vi "ShooterVI.vi"(0 "Shooter Motor 1":T5={"DeviceStatus"={"status"=FALSE, "code"=0, "source"=""}, "Type"=enum."PWM", "PWM"={"PWM Channel"=enum."PWM 1", "DeadBand"={"Name"="", "maxPositivePwm"=0, "minPositivePwm"=0, "centerPwm"=0, "maxNegativePwm"=0, "minNegativePwm"=0, "angularRange"=0}}, "CAN"={"Device Number"=0, "Control Mode"=enum."Percent VBus", "Semaphore"=refnum, "Max Vout"=12.0, "TalonSRX Control Mode"=enum."Percent VBus"}, "Invert"=FALSE}, 2 "ShooterSolenoid":T3={"DevStatus"={"status"=FALSE, "code"=0, "source"=""}, "Pneumatics Control Module"=0, "Forward Solenoid Channel"=enum."Invalid", "Reverse Solenoid Channel"=enum."Invalid"}, 3 "Roller Angle Motor":T5={"DeviceStatus"={"status"=FALSE, "code"=0, "source"=""}, "Type"=enum."PWM", "PWM"={"PWM Channel"=enum."PWM 1", "DeadBand"={"Name"="", "maxPositivePwm"=0, "minPositivePwm"=0, "centerPwm"=0, "maxNegativePwm"=0, "minNegativePwm"=0, "angularRange"=0}}, "CAN"={"Device Number"=0, "Control Mode"=enum."Percent VBus", "Semaphore"=refnum, "Max Vout"=12.0, "TalonSRX Control Mode"=enum."Percent VBus"}, "Invert"=FALSE}, 5 "Shooter Motor 2":T5={"DeviceStatus"={"status"=FALSE, "code"=0, "source"=""}, "Type"=enum."PWM", "PWM"={"PWM Channel"=enum."PWM 1", "DeadBand"={"Name"="", "maxPositivePwm"=0, "minPositivePwm"=0, "centerPwm"=0, "maxNegativePwm"=0, "minNegativePwm"=0, "angularRange"=0}}, "CAN"={"Device Number"=0, "Control Mode"=enum."Percent VBus", "Semaphore"=refnum, "Max Vout"=12.0, "TalonSRX Control Mode"=enum."Percent VBus"}, "Invert"=FALSE}, 7 "Roller Intake Motor":T5={"DeviceStatus"={"status"=FALSE, "code"=0, "source"=""}, "Type"=enum."PWM", "PWM"={"PWM Channel"=enum."Invalid", "DeadBand"={"Name"="", "maxPositivePwm"=0, "minPositivePwm"=0, "centerPwm"=0, "maxNegativePwm"=0, "minNegativePwm"=0, "angularRange"=0}}, "CAN"={"Device Number"=0, "Control Mode"=enum."Percent VBus", "Semaphore"=refnum, "Max Vout"=12.0, "TalonSRX Control Mode"=enum."Percent VBus"}, "Invert"=FALSE}, 9 "Ball Detector Photoeye":T1, 11 "ShooterAngleMotor":T5={"DeviceStatus"={"status"=FALSE, "code"=0, "source"=""}, "Type"=enum."PWM", "PWM"={"PWM Channel"=enum."PWM 1", "DeadBand"={"Name"="", "maxPositivePwm"=0, "minPositivePwm"=0, "centerPwm"=0, "maxNegativePwm"=0, "minNegativePwm"=0, "angularRange"=0}}, "CAN"={"Device Number"=0, "Control Mode"=enum."Percent VBus", "Semaphore"=refnum, "Max Vout"=12.0, "TalonSRX Control Mode"=enum."Percent VBus"}, "Invert"=FALSE}, 12 "Halo Photoeye":T1, 13 "BallHolderSolenoid":T3={"DevStatus"={"status"=FALSE, "code"=0, "source"=""}, "Pneumatics Control Module"=0, "Forward Solenoid Channel"=enum."Invalid", "Reverse Solenoid Channel"=enum."Invalid"}) -> ()   [LabVIEW 2015]
doc: "This VI controls the shooter, roller intake arm, and shooter angle. It recieves motor references as inputs and runs code in single 100 milisecond metronome loop. Sets PID gains for four PID control loops (two shooter motors, roller intake height, and shooter angle). Runs four state machines, controling the shooter wheels as well as shooter plunger and ball position maintance circle, roller intake position, roller intake PID gains, and shooter angle position."
uses:
  <vilib>/Rock Robotics/WPI/MotorControl/WPI_MotorControlDeviceRef.ctl
  <vilib>/Rock Robotics/WPI/MotorControl/WPI_MotorControlType.ctl
  <vilib>/Rock Robotics/SystemInterfaces/DIO/FPGA_DIOPWMChannel.ctl
  <vilib>/Rock Robotics/WPI/PWM/WPI_PWMDeadband.ctl
  <vilib>/Rock Robotics/WPI/CAN/Jaguar/SubVIs/WPI_CANJaguar_ControlMode.ctl
  <vilib>/Rock Robotics/WPI/CAN/TalonSRX/WPI_CANTalonSRX_APIControlMode.ctl
  <vilib>/Rock Robotics/WPI/DigitalInput/WPI_DigitalInputDevRef.ctl
  <vilib>/Rock Robotics/SystemInterfaces/DIO/FPGA_DIOChannel.ctl
  <vilib>/Rock Robotics/WPI/Solenoid/WPI_SolenoidDevRef.ctl
  <vilib>/Rock Robotics/WPI/Solenoid/WPI_SolenoidChannel.ctl
  <vilib>/Rock Robotics/WPI/DriverStation/WPI_DriverStationRobotMode2.ctl
  <vilib>/Rock Robotics/WPI/Solenoid/WPI_SolenoidValue.ctl
  Team Code/Robot Global Data.vi
  <vilib>/Rock Robotics/Network Tables/NT Write Boolean.vi
  <vilib>/Rock Robotics/WPI/Solenoid/WPI_SolenoidSetEnum.vi
panel:
  in  "Wonder Arm I-Zone 2":dbl=20000.0
  in  "Wonder Arm I 2":dbl=0.0001
  in  "Wonder Arm F 2":dbl
  in  "Wonder Arm D 2":dbl
  in  "Wonder Arm P 2":dbl=0.05
  in  "Wonder Arm Vision Position":dbl=50.0
  in  "Shooter Wheel Gear Ratio":dbl=1.375
  in  "Low Goal Wheel Speed":dbl=-3000.0
  in  "Suck Wheel Speed":dbl=2500.0
  in  "Bumper Shot Wheel Speed":dbl=-3250.0
  in  "High Goal Wheel Speed":dbl=-4500.0
  out "Wonder Arm Angle Throttle":dbl
  in  "Pickup Ball Shooter Angle\n(Competition Bot)":dbl=37.0
  in  "Bumper Shot Shooter Angle\n(Competition Bot)":dbl=8.0
  in  "Low Goal Shooter Angle\n(Competition Bot)":dbl=30.0
  in  "High Goal Shooter Angle\n(Competition Bot)":dbl=17.0
  in  "Shooter Angle Offset":dbl
  in  "Bumper Shot Shooter Angle\n(Practice Bot)":dbl=8.0
  in  "Pickup Ball Shooter Angle\n(Practice Bot)":dbl=37.0
  in  "Low Goal Shooter Angle\n(Practice Bot)":dbl=30.0
  in  "High Goal Shooter Angle\n(Practice Bot)":dbl=17.0
  in  "Wonder Arm Low Bar Position":dbl=60.0
  in  "Wonder Arm Down Position":dbl=58.0
  in  "Wonder Arm Pickup Ball Position":dbl=45.0
  in  "Wonder Arm Up Position":dbl
  out "Shooter Angle Throttle":dbl
  in  "Wonder Arm I-Zone":dbl
  in  "Wonder Arm I":dbl
  in  "Wonder Arm F":dbl
  in  "Wonder Arm D":dbl
  in  "Wonder Arm P":dbl=0.01
  out "Shooter Angle Encoder Value":dbl
  out "Shooter Angle Sensor Position":dbl
  in  "Shooter Angle I-Zone":dbl=4000.0
  in  "Shooter Angle I":dbl=1e-06
  in  "Shooter Angle F":dbl
  in  "Shooter Angle D":dbl
  in  "Shooter Angle P":dbl=1.0
  in  "Shooter Motor 2 I-Zone":dbl=70.0
  in  "Shooter Motor 2 I":dbl=0.0006
  in  "Shooter Motor 2 F":dbl=1.35
  in  "Shooter Motor 2 D":dbl
  in  "Shooter Motor 2 P":dbl=9.0
  in  "Shooter Motor 1 I-Zone":dbl=70.0
  in  "Shooter Motor 1 I":dbl=0.0006
  in  "Shooter Motor 1 F":dbl=1.35
  in  "Shooter Motor 1 D":dbl
  in  "Shooter Motor 1 P":dbl=9.0
  in  "error in":errorcluster
  out "Shooter Motor 1 RPM":dbl
  out "Shooter Motor 1 Applied Throttle":dbl
  out "Shooter Motor 2 Applied Throttle":dbl
  # "Shooter Wheels"
  # "Wonder Arm"
  # "Shooter Angle"
  # "Refnum Inputs"
  # "Competition Bot"
  # "Practice Bot"
  # "1 Rotation = 10 Inches from Defense\nHits low bar = Add 2 Rotations\nHits goal High = lower two Rotations"
  # "PID Values"
  # "Shooter Motor 1"
  # "Shooter Motor 2"
  # "Wonder Arm"
  # "Shooter Angle"
  # "High gol native units:\n436"
  # "290.8"
  # "Desired -2181.82\nActual: 1980"
  # "264"
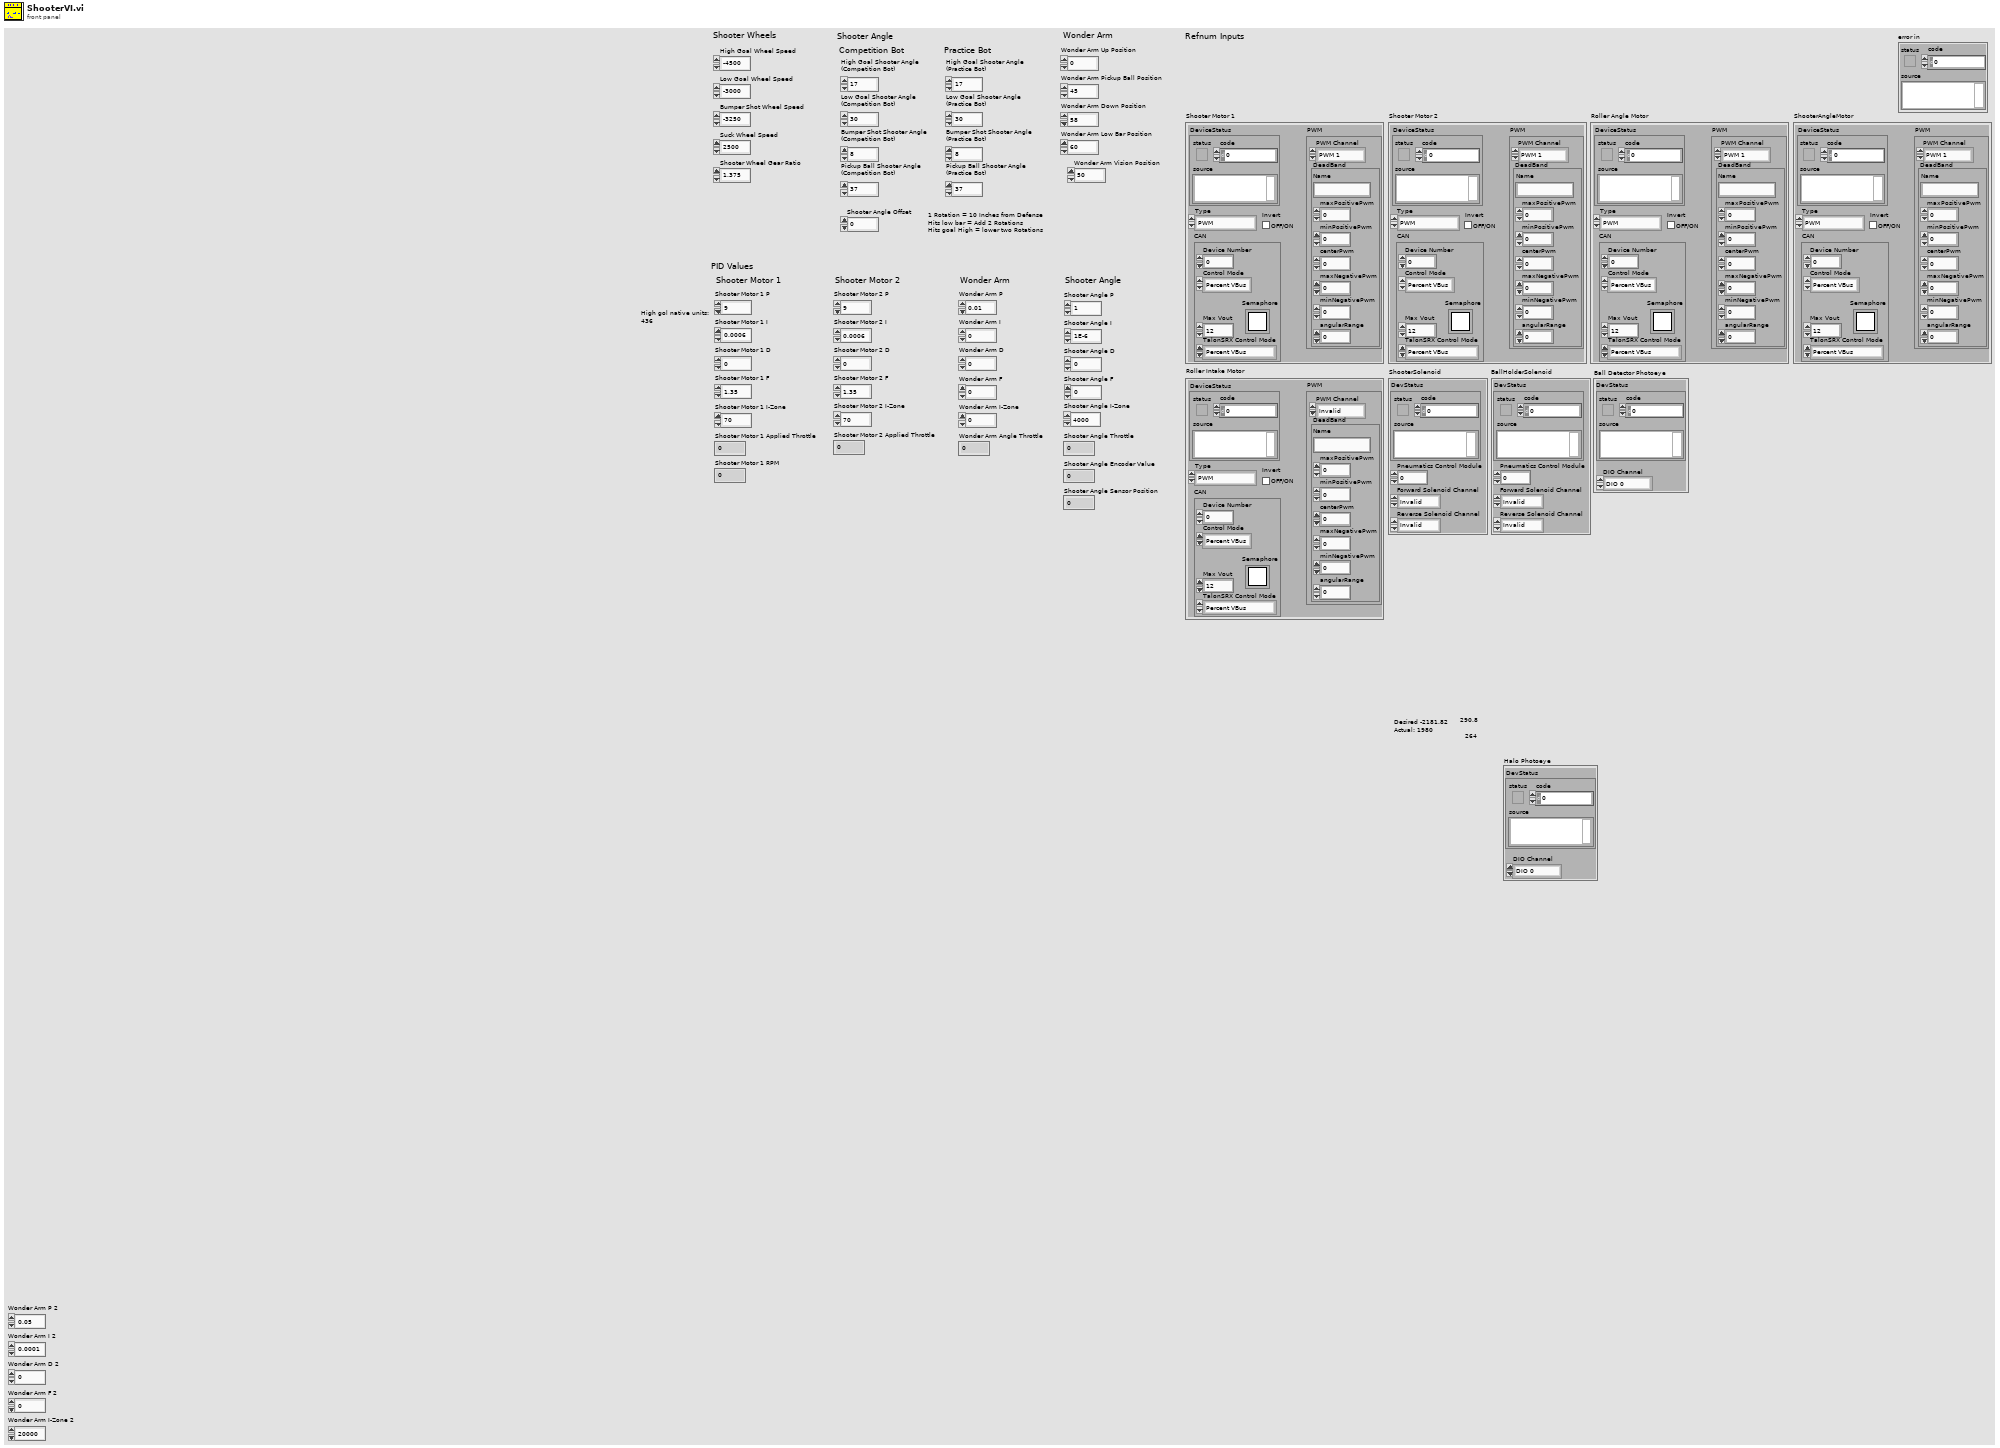
[diagram p1: front panel]
types:
  T1 = typedef "WPI_DigitalInputDevRef.ctl" = cluster{"DevStatus":errorcluster, "DIO Channel":T2}
  T2 = typedef "FPGA_DIOChannel.ctl" = enum8{"DIO 0", "DIO 1", "DIO 2", "DIO 3", "DIO 4", "DIO 5", "DIO 6", "DIO 7", "DIO 8", "DIO 9", "DIO MXP 0", "DIO MXP 1", "DIO MXP 2", "DIO MXP 3", "DIO MXP 4", "DIO MXP 5", "DIO MXP 6", "DIO MXP 7", "DIO MXP 8", "DIO MXP 9", "DIO MXP 10", "DIO MXP 11", "DIO MXP 12", "DIO MXP 13", "DIO MXP 14", "DIO MXP 15", "Invalid"}
  T3 = typedef "WPI_SolenoidDevRef.ctl" = cluster{"DevStatus":errorcluster, "Pneumatics Control Module":u8, "Forward Solenoid Channel":T4, "Reverse Solenoid Channel":T4}
  T4 = typedef "WPI_SolenoidChannel.ctl" = enum8{"Solenoid 0", "Solenoid 1", "Solenoid 2", "Solenoid 3", "Solenoid 4", "Solenoid 5", "Solenoid 6", "Solenoid 7", "Invalid"}
  T5 = typedef "WPI_MotorControlDeviceRef.ctl" = cluster{"DeviceStatus":errorcluster, "Type":T6, "PWM":cluster{"PWM Channel":T7, "DeadBand":T8}, "CAN":cluster{"Device Number":u8, "Control Mode":T9, "Semaphore":T10, "Max Vout":dbl, "TalonSRX Control Mode":T11}, "Invert":bool}
  T6 = typedef "WPI_MotorControlType.ctl" = enum16{"PWM", "CAN", "CANTalonSRX"}
  T7 = typedef "FPGA_DIOPWMChannel.ctl" = enum8{"PWM 0", "PWM 1", "PWM 2", "PWM 3", "PWM 4", "PWM 5", "PWM 6", "PWM 7", "PWM 8", "PWM 9", "PWM MXP 0", "PWM MXP 1", "PWM MXP 2", "PWM MXP 3", "PWM MXP 4", "PWM MXP 5", "PWM MXP 6", "PWM MXP 7", "PWM MXP 8", "PWM MXP 9", "Invalid"}
  T8 = typedef "WPI_PWMDeadband.ctl" = cluster{"Name":string, "maxPositivePwm":i32, "minPositivePwm":i32, "centerPwm":i32, "maxNegativePwm":i32, "minNegativePwm":i32, "angularRange":u16}
  T9 = typedef "WPI_CANJaguar_ControlMode.ctl" = enum8{"Percent VBus", "Current", "Speed", "Position", "Voltage"}
  T10 = typedef "Semaphore RefNum" = refnum<k1>
  T11 = typedef "WPI_CANTalonSRX_APIControlMode.ctl" = enum8{"Percent VBus", "Speed", "Position", "Slave", "Unchanged / Invalid", "Voltage Compensation", "Current", "Motion Profile"}
  T12 = enum16{"ResetBack", "EmergencyManualControl", "ResetForward", "Hold", "Reset", "ManualControl"}
  T13 = enum16{"ResetBack", "ResetForward", "Reset", "Hold", "HighGoal", "LowGoal", "BumperShot", "EmergencyManualControl"}
  T14 = enum16{"Empty", "Suck", "Hold", "LowGoal", "HighGoal", "BumperShot", "Shoot", "Dwell"}
  T15 = cluster{"Wonder Arm P":dbl, "Wonder Arm I":dbl, "Wonder Arm D":dbl, "Wonder Arm F":dbl, "Wonder Arm I-Zone":dbl}
  T16 = typedef "WPI_DriverStationRobotMode2.ctl" = enum16{"Autonomous Disabled", "Autonomous Enabled", "Teleop Disabled", "Teleop Enabled", "Disconnected", "Finish", "Test Disabled", "Test Enabled", "Emergency Stopped"}
  T17 = enum16{"Empty", "Suck", "Hold", "LowGoal", "HighGoal", "Shoot", "Dwell"}
  T18 = typedef "WPI_SolenoidValue.ctl" = enum16{"Off", "On", "Forward", "Reverse"}
  T19 = typedef "WPI_CANTalonSRX_GlobalStatus.ctl" = cluster{"Applied Throttle":dbl, "Module Enabled":bool, "CAN Error":errorcluster, "Closed Loop Error":dbl, "Forward Limit Switch Closed":bool, "Reverse Limit Switch Closed":bool, "Sensor Position":dbl, "Sensor Velocity":dbl, "Current":dbl, "Sticky Fault - Over Temp":bool, "Sticky Fault - Under Voltage":bool, "Sticky Fault - Forward Limit":bool, "Sticky Fault - Reverse Limit":bool, "Sticky Fault - Forward Soft Limit":bool, "Sticky Fault - Reverse Soft Limit":bool, "Brake is Enabled":bool, "Encoder Position":dbl, "Encoder Velocity":dbl, "Encoder Index Count":dbl, "Encoder A Pin State":bool, "Encoder B Pin State":bool, "Encoder Index Pin State":bool, "Analog In":dbl, "Analog In Velocity":dbl, "Temperature (C)":dbl, "Battery Voltage":dbl, "Control 5 Is Supported":bool, "Current Profile Slot Select":dbl, "Pos Div 8":bool, "Vel Div 4":bool, "Pulse Width Position":i32, "Pulse Width Velocity":i32, "Pulse Width Rise To Rise (us)":i32, "Pulse Width Rise To Fall (us)":i32, "Mot Prof Active Is Under Run":bool, "Mot Prof Active Has Under Run":bool, "Mot Prof Active Is Last":bool, "Mot Prof Active Velocity Only":bool, "Mot Prof Active Is Valid":bool, "Mot Prof Buffer Is Full":bool, "Mot Prof Active Profile Slot Select":i32, "Mot Prof NextID":i32, "Mot Prof Count":i32, "Mot Prof Active Velocity":dbl, "Mot Prof Active Position":dbl, "Mot Prof Output Enable":i32}
  T20 = cluster{"Wonder Arm P 2":dbl, "Wonder Arm I 2":dbl, "Wonder Arm D 2":dbl, "Wonder Arm F 2":dbl, "Wonder Arm I-Zone 2":dbl}
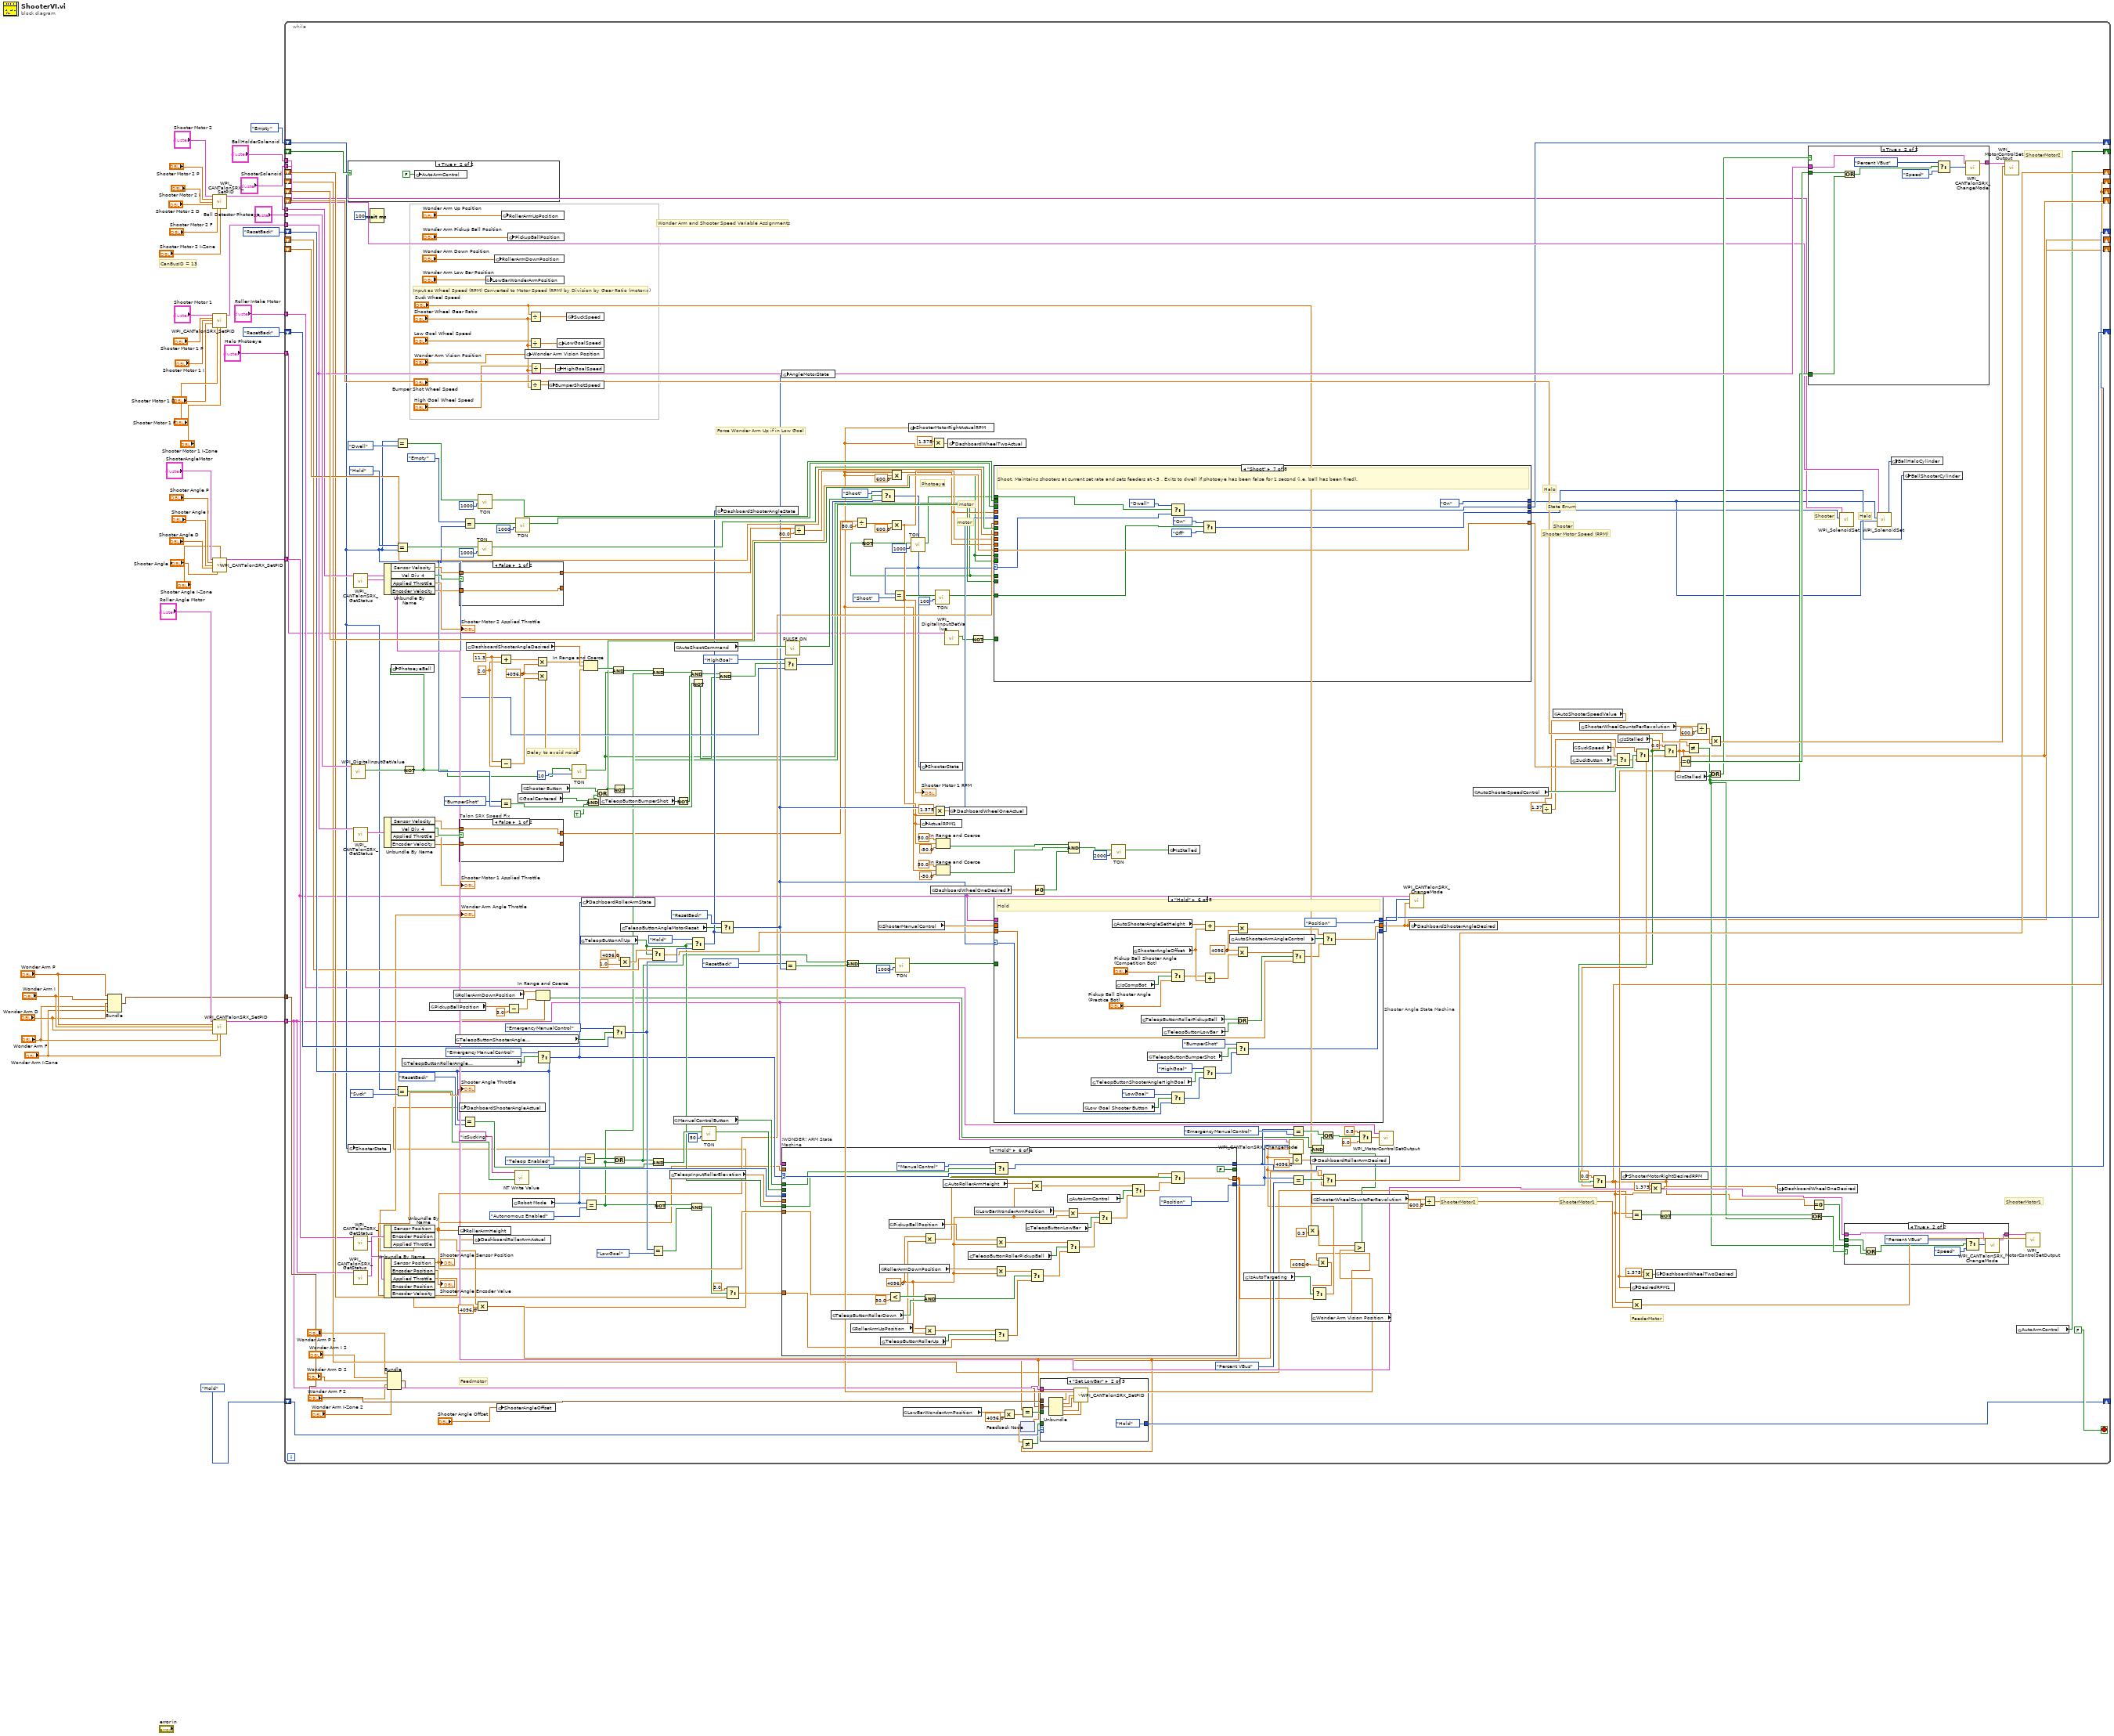
[diagram p0: block diagram]
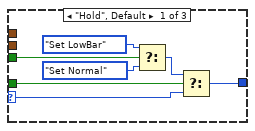
[diagram p2: hidden frame]
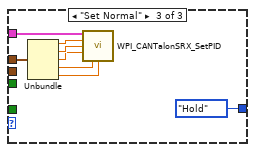
[diagram p3: hidden frame]
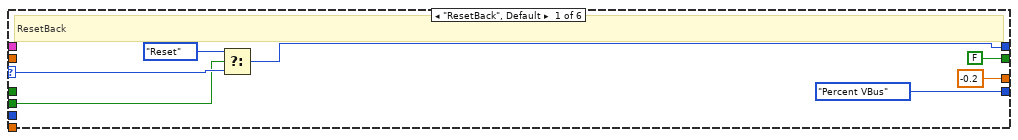
[diagram p5: hidden frame]
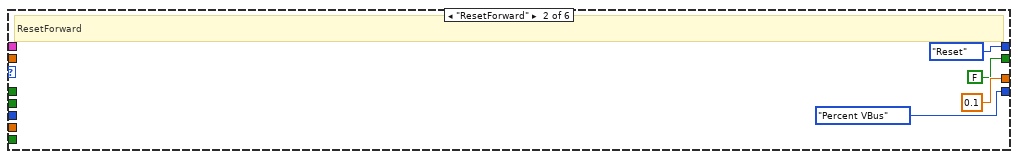
[diagram p6: hidden frame]
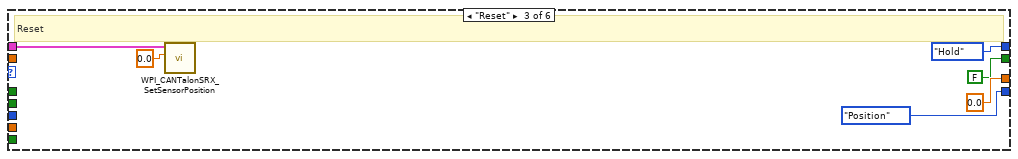
[diagram p7: hidden frame]
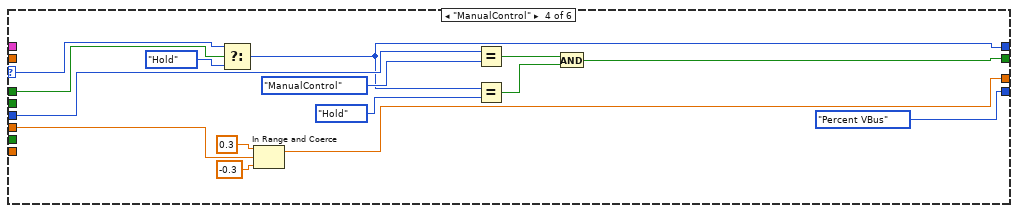
[diagram p8: hidden frame]
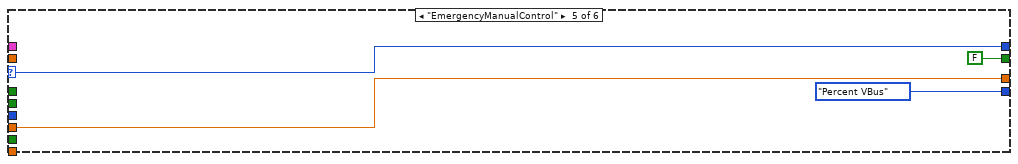
[diagram p9: hidden frame]
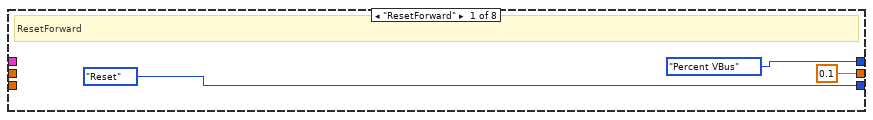
[diagram p10: hidden frame]
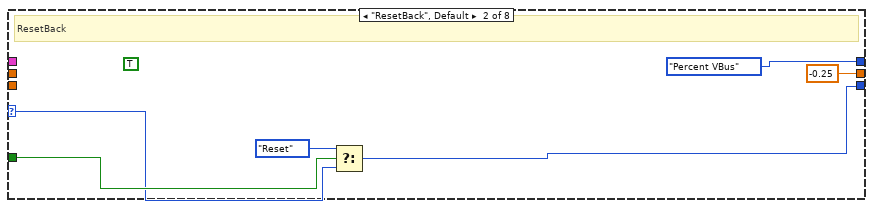
[diagram p11: hidden frame]
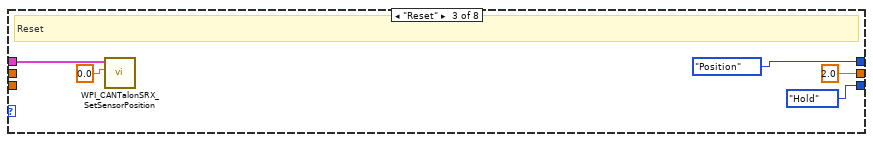
[diagram p12: hidden frame]
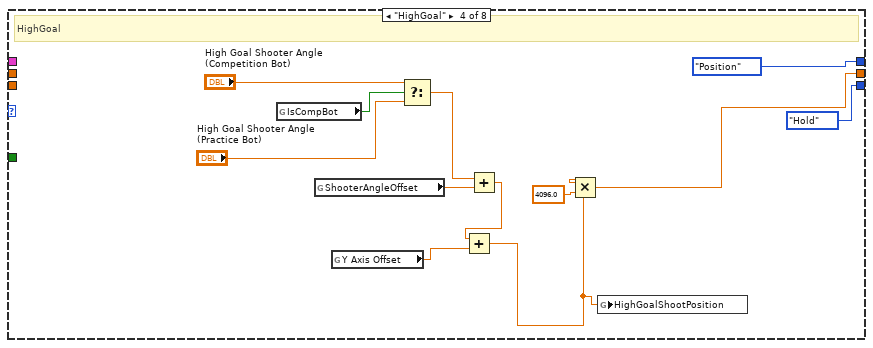
[diagram p13: hidden frame]
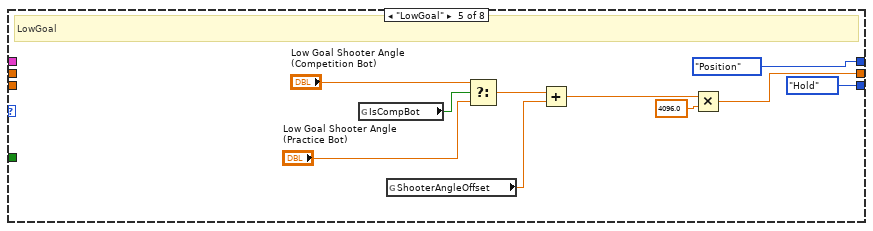
[diagram p14: hidden frame]
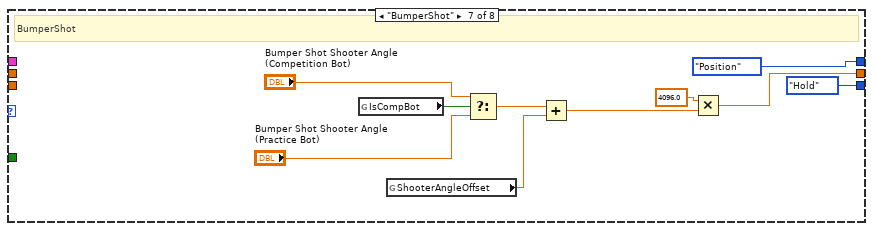
[diagram p15: hidden frame]
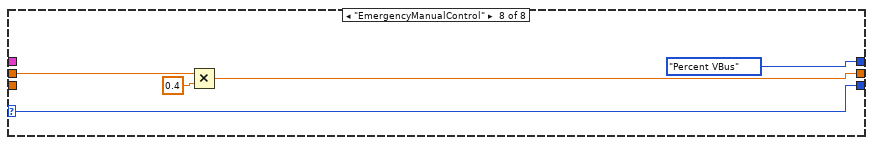
[diagram p16: hidden frame]
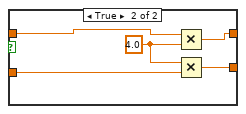
[diagram p19: hidden frame]
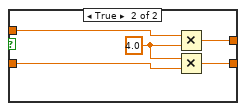
[diagram p20: hidden frame]
diagram:
  # "CanBusID = 13"
  n1 = Bundle("Wonder Arm P"="Wonder Arm P", "Wonder Arm I"="Wonder Arm I", "Wonder Arm D"="Wonder Arm D", "Wonder Arm F"="Wonder Arm F", "Wonder Arm I-Zone"="Wonder Arm I-Zone") -> (w2:T15)  [unwired: 1 in]
  n2 = call <vilib>:"WPI_CANTalonSRX_SetPID.vi"("CAN Talon SRX Ref"="Shooter Motor 2", "P"="Shooter Motor 2 P", "I"="Shooter Motor 2 I", "D"="Shooter Motor 2 D", "F"="Shooter Motor 2 F", "I Zone"="Shooter Motor 2 I-Zone") -> ("CAN Talon SRX Ref"=w35:T5)  [unwired: 8 in, 1 out]
  n3 = call <vilib>:"WPI_CANTalonSRX_SetPID.vi"("CAN Talon SRX Ref"="Shooter Motor 1", "P"="Shooter Motor 1 P", "I"="Shooter Motor 1 I", "D"="Shooter Motor 1 D", "F"="Shooter Motor 1 F", "I Zone"="Shooter Motor 1 I-Zone") -> ("CAN Talon SRX Ref"=w33:T5)  [unwired: 8 in, 1 out]
  n4 = call <vilib>:"WPI_CANTalonSRX_SetPID.vi"("CAN Talon SRX Ref"="ShooterAngleMotor", "P"="Shooter Angle P", "I"="Shooter Angle I", "D"="Shooter Angle D", "F"="Shooter Angle F", "I Zone"="Shooter Angle I-Zone") -> ("CAN Talon SRX Ref"=w17:T5)  [unwired: 8 in, 1 out]
  n5 = call <vilib>:"WPI_CANTalonSRX_SetPID.vi"("CAN Talon SRX Ref"="Roller Angle Motor", "P"="Wonder Arm P", "I"="Wonder Arm I", "D"="Wonder Arm D", "F"="Wonder Arm F", "I Zone"="Wonder Arm I-Zone") -> ("CAN Talon SRX Ref"=w14:T5)  [unwired: 8 in, 1 out]
  n6 = while {
    tunnel: w33 -> [w273]
    tunnel: w35 -> [w276]
    tunnel: "Ball Detector Photoeye" -> [w302]
    shift-right: [w87] -> _
    shift-left: _ -> [w299]
    shift-right: [w90] -> _
    shift-left: _ -> [w280]
    shift-right: [w90] -> _
    shift-left: _ -> [w191]
    shift-right: [w87] -> _
    shift-left: _ -> [w53]
    tunnel: w17 -> [w147]
    shift-right: [w40] -> _
    shift-left: _ -> [w217]
    shift-right: [w70] -> _
    shift-left: T14."Empty" -> [w155]
    tunnel: w14 -> [w76]
    shift-right: [w261] -> _
    shift-left: _ -> [w225]
    shift-right: [w236] -> _
    shift-left: T12."ResetBack" -> [w237]
    shift-right: [w259] -> _
    shift-left: T13."ResetBack" -> [w257]
    tunnel: "Roller Intake Motor" -> [w188]
    tunnel: "ShooterSolenoid" -> [w68]
    shift-right: [w39] -> _
    shift-left: _ -> [w230]
    tunnel: "BallHolderSolenoid" -> [w108]
    shift-right: [w78] -> _
    shift-left: enum16{"Hold", "Set LowBar", "Set Normal"}."Hold" -> [w73]
    tunnel: w2 -> [w77]
    tunnel: "Halo Photoeye" -> [w71]
    stop <- FALSE stop-if-true
    w192 = 2.0 ("y")
    w207 = 4096.0 ("y")
    w193 = 11.3 ("x")
    # "Input as Wheel Speed (RPM) Converted to Motor Speed (RPM) by Division by Gear Ratio (motor:x)"
    # "Wonder Arm and Shooter Speed Variable Assignments"
    # "Shooter Motor Speed (RPM)"
    # "State Enum"
    # "Shooter"
    # "Halo"
    # "Halo"
    # "Shooter"
    # "motor"
    # "motor"
    # "Force Wonder Arm Up if in Low Goal"
    # "Photoeye"
    # "FeederMotor"
    # "ShooterMotor2"
    # "ShooterMotor1"
    # "Feedmotor"
    # "Delay to avoid noise"
    # "ShooterMotor2"
    # "ShooterMotor1"
    n7 = case shown="True" w230 {
      frame False {
      }
      frame True {
        n8 = global write "Robot Global Data.vi" "AutoArmControl"(FALSE ("AutoArmControl")) -> ()
      }
    }
    n9 = global write "Robot Global Data.vi" "ShooterState"(w155) -> ()
    n10 = call <vilib>:"WPI_DigitalInputGetValue.vi"("DigitalInputDevRef"=w302) -> ("Value"=w289:bool)  [unwired: 8 in, 2 out]
    n11 = call <vilib>:"WPI_CANTalonSRX_GetStatus.vi"("CAN Talon SRX Ref"=w276) -> ("Talon SRX Status"=w300:T19)  [unwired: 8 in, 2 out]
    n12 = call <vilib>:"WPI_CANTalonSRX_GetStatus.vi"("CAN Talon SRX Ref"=w273) -> ("Talon SRX Status"=w301:T19)  [unwired: 8 in, 2 out]
    n13 = call <vilib>:"WPI_CANTalonSRX_GetStatus.vi"("CAN Talon SRX Ref"=w147) -> ("Talon SRX Status"=w269:T19)  [unwired: 8 in, 2 out]
    n14 = call <vilib>:"WPI_CANTalonSRX_GetStatus.vi"("CAN Talon SRX Ref"=w76) -> ("Talon SRX Status"=w262:T19)  [unwired: 8 in, 2 out]
    n15 = Wait (ms)(milliseconds to wait=u32 100) -> ()  [unwired: 1 out]
    n16 = Unbundle By Name(w300) -> ("Sensor Velocity"=w177:dbl, "Vel Div 4"=w296:bool, "Applied Throttle"=→"Shooter Motor 2 Applied Throttle":dbl, "Encoder Velocity"=w172:dbl)
    n17 = Unbundle By Name(w301) -> ("Sensor Velocity"=w178:dbl, "Vel Div 4"=w297:bool, "Applied Throttle"=→"Shooter Motor 1 Applied Throttle":dbl, "Encoder Velocity"=w173:dbl)
    n18 = Unbundle By Name(w262) -> ("Sensor Position"=w119:dbl, "Applied Throttle"=→"Wonder Arm Angle Throttle":dbl)  [unwired: 1 out]
    n19 = Unbundle By Name(w269) -> ("Sensor Position"=w159:dbl, "Encoder Position"=→"Shooter Angle Encoder Value":dbl, "Applied Throttle"=→"Shooter Angle Throttle":dbl, "Encoder Position"=w41:dbl)  [unwired: 1 out]
    "Shooter Angle Sensor Position" <- w159
    n20 = Bundle("Wonder Arm P 2"="Wonder Arm P 2", "Wonder Arm I 2"="Wonder Arm I 2", "Wonder Arm D 2"="Wonder Arm D 2", "Wonder Arm F 2"="Wonder Arm F 2", "Wonder Arm I-Zone 2"="Wonder Arm I-Zone 2") -> (w42:T20)  [unwired: 1 in]
    n21 = Equal?(x=w155, y=T14."Dwell") -> (x = y?=w295:bool)
    n22 = Equal?(x=T17."Hold", y=w155) -> (x = y?=w283:bool)
    n23 = Equal?(x=w155, y=T14."Suck") -> (x = y?=w197:bool)
    n24 = Not(x=w289) -> (.not. x?=w109:bool)
    n25 = global write "Robot Global Data.vi" "PhotoeyeBall"(w109) -> ()
    n26 = global read "Robot Global Data.vi" "TeleopButtonRollerAngle\nEmergencyManual"() -> (w264:bool)
    n27 = global read "Robot Global Data.vi" "PickupBallPosition"() -> (w240:dbl)
    n28 = global read "Robot Global Data.vi" "RollerArmDownPosition"() -> (w238:dbl)
    n29 = global read "Robot Global Data.vi" "TeleopButtonShooterAngle\nEmergencyManual"() -> (w258:bool)
    n30 = global write "Robot Global Data.vi" "RollerArmHeight"(w119) -> ()
    n31 = case shown="False" w296 {
      tunnel: w177 -> [w499 w504]
      tunnel: [w499 w503] -> w125
      tunnel: [w498 w501] -> _
      tunnel: w172 -> [w498 w500]
      frame False {
      }
      frame True {
        w502 = 4.0 ("y")
        n32 = Multiply(x=w504, y=w502) -> (x*y=w503:dbl)
        n33 = Multiply(x=w502, y=w500) -> (x*y=w501:dbl)
      }
    }
    n34 = case "Talon SRX Speed Fix" shown="False" w297 {
      tunnel: w178 -> [w506 w511]
      tunnel: [w506 w510] -> w121
      tunnel: [w505 w509] -> _
      tunnel: w173 -> [w505 w507]
      frame False {
      }
      frame True {
        w508 = 4.0 ("y")
        n35 = Multiply(x=w511, y=w508) -> (x*y=w510:dbl)
        n36 = Multiply(x=w508, y=w507) -> (x*y=w509:dbl)
      }
    }
    n37 = global write "Robot Global Data.vi" "DashboardShooterAngleActual"(w41) -> ()
    n38 = Equal?(x=T17."Empty", y=w155) -> (x = y?=w287:bool)
    n39 = Equal?(x=w237, y=T12."ResetBack") -> (x = y?=w200:bool)
    n40 = global read "Robot Global Data.vi" "DashboardShooterAngleDesired"() -> (w210:dbl)
    n41 = global write "Robot Global Data.vi" "DashboardRollerArmActual"(w119) -> ()
    n42 = Multiply(x=w119, y=4096.0) -> (x*y=w145:dbl)
    n43 = call "TON.vi"("Delay (ms)"=u32 1000, "Input"=w295) -> ("Output"=w294:bool)  [unwired: 9 in]
    n44 = call "TON.vi"("Delay (ms)"=u32 1000, "Input"=w283) -> ("Output"=w281:bool)  [unwired: 9 in]
    n45 = global write "Robot Global Data.vi" "LowBarWonderArmPosition"("Wonder Arm Low Bar Position") -> ()
    n46 = global write "Robot Global Data.vi" "RollerArmDownPosition"("Wonder Arm Down Position") -> ()
    n47 = global write "Robot Global Data.vi" "ShooterAngleOffset"("Shooter Angle Offset") -> ()
    n48 = Add(x=w193, y=w192) -> (x+y=w209:dbl)
    n49 = Subtract(x=w193, y=w192) -> (x-y=w206:dbl)
    n50 = Equal?(x=T14."BumperShot", y=w155) -> (x = y?=w153:bool)
    n51 = global write "Robot Global Data.vi" "RollerArmUpPosition"("Wonder Arm Up Position") -> ()
    n52 = Subtract(x=w240, y=3.0) -> (x-y=w239:dbl)
    n53 = global write "Robot Global Data.vi" "PickupBallPosition"("Wonder Arm Pickup Ball Position") -> ()
    n54 = global read "Robot Global Data.vi" "Robot Mode"() -> (w229:T16)
    n55 = call-poly <vilib>:"NT Write Value.vi"("Boolean"=w197, "Name"="isSucking") -> ()  [unwired: 9 in, 1 out]
    n56 = call "TON.vi"("Delay (ms)"=u32 1000, "Input"=w287) -> ("Output"=w285:bool)  [unwired: 9 in]
    n57 = global read "Robot Global Data.vi" "GoalCentered"() -> (w107:bool)
    n58 = global read "Robot Global Data.vi" "Shooter Button"() -> (w106:bool)
    n59 = global write "Robot Global Data.vi" "Wonder Arm Vision Position"("Wonder Arm Vision Position") -> ()
    n60 = Divide(x="Suck Wheel Speed", y="Shooter Wheel Gear Ratio") -> (x/y=w144:dbl)
    n61 = Divide(x="Low Goal Wheel Speed", y="Shooter Wheel Gear Ratio") -> (x/y=w143:dbl)
    n62 = Divide(x="Bumper Shot Wheel Speed", y="Shooter Wheel Gear Ratio") -> (x/y=w142:dbl)
    n63 = Divide(x="High Goal Wheel Speed", y="Shooter Wheel Gear Ratio") -> (x/y=w141:dbl)
    n64 = Multiply(x=w209, y=w207) -> (x*y=w208:dbl)
    n65 = Multiply(x=w207, y=w206) -> (x*y=w205:dbl)
    n66 = In Range and Coerce(upper limit=w238, x=w119, lower limit=w239) -> (In Range?=w114:bool)  [unwired: 1 out]
    n67 = Select(t=T12."EmergencyManualControl", s=w264, f=w237) -> (s? t:f=w212:T12)
    n68 = global write "Robot Global Data.vi" "BumperShotSpeed"(w142) -> ()
    n69 = global write "Robot Global Data.vi" "HighGoalSpeed"(w141) -> ()
    n70 = global write "Robot Global Data.vi" "LowGoalSpeed"(w143) -> ()
    n71 = global write "Robot Global Data.vi" "SuckSpeed"(w144) -> ()
    n72 = call "TON.vi"("Delay (ms)"=u32 10, "Input"=w109) -> ("Output"=w58:bool)  [unwired: 9 in]
    n73 = global read "Robot Global Data.vi" "TeleopButtonAllUp"() -> (w214:bool)
    n74 = global write "Robot Global Data.vi" "DashboardRollerArmState"(w212) -> ()
    n75 = Equal?(x=w229, y=WPI_DriverStationRobotMode2."Teleop Enabled") -> (x = y?=w228:bool)
    n76 = In Range and Coerce(upper limit=w208, x=w210, lower limit=w205) -> (In Range?=w204:bool)  [unwired: 1 out]
    n77 = Equal?(x=w229, y=WPI_DriverStationRobotMode2."Autonomous Enabled") -> (x = y?=w149:bool)
    n78 = And(x=w107, y=TRUE) -> (x .and. y?=w104:bool)
    n79 = Or(x=w106, y=w104) -> (x .or. y?=w105:bool)
    n80 = global read "Robot Global Data.vi" "TeleopButtonBumperShot"() -> (w194:bool)
    n81 = And(x=w204, y=w58) -> (x .and. y?=w203:bool)
    n82 = Select(t=T13."EmergencyManualControl", s=w258, f=w257) -> (s? t:f=w219:T13)
    n83 = Not(x=w105) -> (.not. x?=w202:bool)
    n84 = Or(x=w228, y=w149) -> (x .or. y?=w163:bool)
    n85 = Multiply(x=4096.0, y=1.0) -> (x*y=w222:dbl)
    n86 = global read "Robot Global Data.vi" "TeleopButtonAngleMotorReset"() -> (w183:bool)
    n87 = Select(t=w222, s=w214, f=w217) -> (s? t:f=w216:dbl)
    n88 = Equal?(x=w219, y=T13."LowGoal") -> (x = y?=w157:bool)
    n89 = And(x=w203, y=w202) -> (x .and. y?=w196:bool)
    n90 = And(x=w163, y=w200) -> (x .and. y?=w243:bool)
    n91 = Not(x=w149) -> (.not. x?=w156:bool)
    n92 = global read "Robot Global Data.vi" "TeleopInputRollerElevation"() -> (w265:dbl)
    n93 = global read "Robot Global Data.vi" "ManualControlButton"() -> (w260:bool)
    n94 = global read "Robot Global Data.vi" "AutoShootCommand"() -> (w168:bool)
    n95 = Not(x=w194) -> (.not. x?=w195:bool)
    n96 = And(x=w196, y=w195) -> (x .and. y?=w151:bool)
    n97 = And(x=w156, y=w157) -> (x .and. y?=w158:bool)
    n98 = Not(x=w153) -> (.not. x?=w152:bool)
    n99 = Select(t=T13."Hold", s=w214, f=w219) -> (s? t:f=w213:T13)
    n100 = call "TON.vi"("Delay (ms)"=u32 50, "Input"=w243) -> ("Output"=w246:bool)  [unwired: 9 in]
    n101 = global write "Robot Global Data.vi" "DashboardShooterAngleState"(w213) -> ()
    n102 = And(x=w151, y=w152) -> (x .and. y?=w150:bool)
    n103 = Select(t=T13."ResetBack", s=w183, f=w213) -> (s? t:f=w166:T13)
    n104 = Select(t=3.0 ("y"), s=w158, f=w225) -> (s? t:f=w224:dbl)
    n105 = global write "Robot Global Data.vi" "AngleMotorState"(w166) -> ()
    n106 = case "!WONDER! ARM State Machine" shown="\"Hold\"" w212 {
      selector: w212 -> [w335 _ _ w355 w362 w392]
      tunnel: [w334 T12."Reset" T12."Hold" w350 w362 w391] -> w236
      tunnel: [WPI_CANTalonSRX_APIControlMode."Percent VBus" ("Control Mode") WPI_CANTalonSRX_APIControlMode."Percent VBus" ("Control Mode") WPI_CANTalonSRX_APIControlMode."Position" ("Control Mode") WPI_CANTalonSRX_APIControlMode."Percent VBus" ("Control Mode") WPI_CANTalonSRX_APIControlMode."Percent VBus" ("Control Mode") WPI_CANTalonSRX_APIControlMode."Position" ("Control Mode")] -> w235
      tunnel: [-0.2 ("Output") 0.1 ("Output") 0.0 ("Output") w356 w361 w368] -> w74
      tunnel: w265 -> [_ _ _ w357 w361 _]
      tunnel: w224 -> [_ _ _ _ _ w394]
      tunnel: w119 -> [_ _ _ _ _ _]
      tunnel: [FALSE FALSE FALSE w346 FALSE FALSE] -> _
      tunnel: w260 -> [_ _ _ w347 _ w389]
      tunnel: w76 -> [_ _ w340 _ _ _]
      tunnel: w246 -> [w329 _ _ _ _ _]
      tunnel: w237 -> [_ _ _ w353 _ _]
      tunnel: w159 -> [_ _ _ _ _ w373]
      tunnel: w214 -> [_ _ _ _ _ w370]
      frame "ResetBack", Default {
        # "ResetBack"
        n107 = Select(t=T12."Reset", s=w329, f=w335) -> (s? t:f=w334:T12)
      }
      frame "ResetForward" {
        # "ResetForward"
      }
      frame "Reset" {
        # "Reset"
        n108 = call <vilib>:"WPI_CANTalonSRX_SetSensorPosition.vi"("New Sensor Position"=0.0, "CAN Talon SRX Ref"=w340) -> ()  [unwired: 8 in, 2 out]
      }
      frame "ManualControl" {
        n109 = Select(t=w355, s=w347, f=T12."Hold") -> (s? t:f=w350:T12)
        n110 = In Range and Coerce(upper limit=0.3, x=w357, lower limit=-0.3) -> (coerced(x)=w356:dbl)  [unwired: 1 out]
        n111 = Equal?(x=w353, y=T12."ManualControl") -> (x = y?=w351:bool)
        n112 = Equal?(x=w350, y=T12."Hold") -> (x = y?=w348:bool)
        n113 = And(x=w351, y=w348) -> (x .and. y?=w346:bool)
      }
      frame "EmergencyManualControl" {
      }
      frame "Hold" {
        w366 = 4096.0 ("y")
        n114 = global read "Robot Global Data.vi" "TeleopButtonRollerDown"() -> (w375:bool)
        n115 = global read "Robot Global Data.vi" "RollerArmUpPosition"() -> (w365:dbl)
        n116 = global read "Robot Global Data.vi" "RollerArmDownPosition"() -> (w384:dbl)
        n117 = global read "Robot Global Data.vi" "TeleopButtonRollerUp"() -> (w397:bool)
        n118 = Less?(x=w373, y=30.0) -> (x < y?=w372:bool)
        n119 = global read "Robot Global Data.vi" "PickupBallPosition"() -> (w385:dbl)
        n120 = Multiply(x=w366, y=w365) -> (x*y=w367:dbl)
        n121 = And(x=w372, y=w375) -> (x .and. y?=w371:bool)
        n122 = Multiply(x=w365, y=w366) -> (x*y=w386:dbl)
        n123 = global read "Robot Global Data.vi" "AutoRollerArmHeight"() -> (w376:dbl)
        n124 = global read "Robot Global Data.vi" "TeleopButtonRollerPickupBall"() -> (w398:bool)
        n125 = global read "Robot Global Data.vi" "LowBarWonderArmPosition"() -> (w381:dbl)
        n126 = Multiply(x=w385, y=w366) -> (x*y=w388:dbl)
        n127 = Multiply(x=w384, y=w366) -> (x*y=w387:dbl)
        n128 = Select(t=T12."ManualControl", s=w389, f=w392) -> (s? t:f=w391:T12)
        n129 = Select(t=w386, s=w397, f=w394) -> (s? t:f=w396:dbl)
        n130 = global read "Robot Global Data.vi" "TeleopButtonLowBar"() -> (w380:bool)
        n131 = Multiply(x=w376, y=w366) -> (x*y=w377:dbl)
        n132 = Select(t=w387, s=w371, f=w396) -> (s? t:f=w395:dbl)
        n133 = Multiply(x=w381, y=w366) -> (x*y=w382:dbl)
        n134 = Select(t=w388, s=w398, f=w395) -> (s? t:f=w383:dbl)
        n135 = global read "Robot Global Data.vi" "AutoArmControl"() -> (w379:bool)
        n136 = Select(t=w382, s=w380, f=w383) -> (s? t:f=w378:dbl)
        n137 = Select(t=w377, s=w379, f=w378) -> (s? t:f=w369:dbl)
        n138 = Select(t=w367, s=w370, f=w369) -> (s? t:f=w368:dbl)
      }
    }
    n139 = Select(t=T14."HighGoal", s=w150, f=w155) -> (s? t:f=w148:T14)
    n140 = Equal?(x=T13."ResetBack", y=w166) -> (x = y?=w164:bool)
    n141 = call "PULSE ON.vi"("Input"=w168) -> ("Output"=w167:bool)  [unwired: 10 in]
    n142 = Divide(x=w125, y=80.0) -> (x/y=w128:dbl)
    n143 = And(x=w163, y=w164) -> (x .and. y?=w161:bool)
    n144 = Divide(x=w121, y=80.0) -> (x/y=w124:dbl)
    n145 = Not(x=w58) -> (.not. x?=w59:bool)
    n146 = global read "Robot Global Data.vi" "ShooterManualControl"() -> (w255:dbl)
    n147 = Select(t=T14."Shoot", s=w167, f=w148) -> (s? t:f=w62:T14)
    n148 = Multiply(x=w128, y=600.0) -> (x*y=w94:dbl)
    n149 = Multiply(x=w124, y=600.0) -> (x*y=w120:dbl)
    "Shooter Motor 1 RPM" <- w120
    n150 = Equal?(x=w62, y=T14."Shoot") -> (x = y?=w63:bool)
    n151 = call "TON.vi"("Delay (ms)"=u32 1000, "Input"=w161) -> ("Output"=w160:bool)  [unwired: 9 in]
    n152 = global read "Robot Global Data.vi" "LowBarWonderArmPosition"() -> (w82:dbl)
    n153 = global write "Robot Global Data.vi" "ShooterMotorRightActualRPM"(w94) -> ()
    n154 = call "TON.vi"("Delay (ms)"=u32 1000, "Input"=w59) -> ("Output"=w57:bool)  [unwired: 9 in]
    n155 = global write "Robot Global Data.vi" "ShooterState"(w62) -> ()
    n156 = global write "Robot Global Data.vi" "ActualRPM1"(w120) -> ()
    n157 = global read "Robot Global Data.vi" "DashboardWheelOneDesired"() -> (w181:dbl)
    n158 = Multiply(x=1.375, y=w94) -> (x*y=w93:dbl)
    n159 = Multiply(x=1.375, y=w120) -> (x*y=w97:dbl)
    n160 = call "TON.vi"("Delay (ms)"=u32 100, "Input"=w63) -> ("Output"=w61:bool)  [unwired: 9 in]
    n161 = In Range and Coerce(upper limit=50.0, x=w120, lower limit=-50.0) -> (In Range?=w55:bool)  [unwired: 1 out]
    n162 = In Range and Coerce(upper limit=50.0, x=w94, lower limit=-50.0) -> (In Range?=w54:bool)  [unwired: 1 out]
    n163 = call <vilib>:"WPI_DigitalInputGetValue.vi"("DigitalInputDevRef"=w71) -> ("Value"=w69:bool)  [unwired: 8 in, 2 out]
    n164 = global write "Robot Global Data.vi" "DashboardWheelTwoActual"(w93) -> ()
    n165 = global write "Robot Global Data.vi" "DashboardWheelOneActual"(w97) -> ()
    n166 = Not(x=w69) -> (.not. x?=w66:bool)
    n167 = case shown="\"Shoot\"" w62 {
      selector: w62 -> [w518 _ w542 w567 w604 w634 w651 w663]
      tunnel: [w517 w523 w529 w561 w598 w629 w656 w662] -> w70
      tunnel: [0.0 w526 0.0 w553 w573 w618 w655 w661] -> w117
      tunnel: w58 -> [_ w521 _ w559 w595 w627 _ _]
      tunnel: w105 -> [_ _ _ w549 w615 w635 _ _]
      tunnel: w120 -> [_ _ _ w548 _ w637 _ _]
      tunnel: w299 -> [_ _ _ _ _ _ w655 w661]
      tunnel: w94 -> [_ _ _ w545 w611 w636 _ _]
      tunnel: w294 -> [_ _ _ _ _ _ _ w660]
      tunnel: w285 -> [w516 _ _ _ _ _ _ _]
      tunnel: w281 -> [_ _ w543 _ _ _ _ _]
      tunnel: w280 -> [_ _ _ _ _ _ _ _]
      tunnel: w105 -> [_ _ _ _ _ _ _ _]
      tunnel: [WPI_SolenoidValue."Off" ("Value") WPI_SolenoidValue."Off" ("Value") WPI_SolenoidValue."Off" ("Value") WPI_SolenoidValue."Off" ("Value") WPI_SolenoidValue."Off" ("Value") WPI_SolenoidValue."Off" ("Value") w650 WPI_SolenoidValue."Off" ("Value")] -> w67
      tunnel: w159 -> [_ _ _ _ w587 _ _ _]
      tunnel: w120 -> [_ _ _ _ w569 _ _ _]
      tunnel: w166 -> [_ _ _ _ w584 _ _ _]
      tunnel: w149 -> [_ _ _ _ _ _ _ _]
      tunnel: [WPI_SolenoidValue."On" ("Value") WPI_SolenoidValue."On" ("Value") WPI_SolenoidValue."Off" ("Value") WPI_SolenoidValue."Off" ("Value") WPI_SolenoidValue."Off" ("Value") WPI_SolenoidValue."Off" ("Value") WPI_SolenoidValue."On" ("Value") WPI_SolenoidValue."On" ("Value")] -> w56
      tunnel: w66 -> [_ w519 _ _ _ _ _ _]
      tunnel: w61 -> [_ _ _ _ _ _ w648 _]
      tunnel: w57 -> [_ _ _ _ _ _ w647 _]
      frame "Empty", Default {
        # "Empty. Default state. No motor Commands. Exits after 1 seconds to Suck case."
        n168 = Select(t=T14."Suck", s=w516, f=w518) -> (s? t:f=w517:T14)
      }
      frame "Suck" {
        # "Suck. Runs feeder motors at .5; shooter motors are commanded -4000 rpm. Exits after photoeye has been true for 0.2 seconds to hold case."
        n169 = And(x=w519, y=w521) -> (x .and. y?=w520:bool)
        n170 = Select(t=T14."Hold", s=w520, f=T14."Suck") -> (s? t:f=w523:T14)
        n171 = global read "Robot Global Data.vi" "SuckSpeed"() -> (w526:dbl)
      }
      frame "Hold" {
        # "Hold. All motors are still to maintain ball. Exits by default after 1 second to LowGoal or to LowGoal or HighGoal if their respective buttons are pressed."
        n172 = global read "Robot Global Data.vi" "Low Goal Shooter Button"() -> (w541:bool)
        n173 = global read "Robot Global Data.vi" "TeleopButtonShooterAngleHighGoal"() -> (w539:bool)
        n174 = Select(t=T14."LowGoal", s=w543, f=w542) -> (s? t:f=w540:T14)
        n175 = global read "Robot Global Data.vi" "TeleopButtonBumperShot"() -> (w532:bool)
        n176 = Select(t=T14."LowGoal", s=w541, f=w540) -> (s? t:f=w538:T14)
        n177 = Select(t=T14."HighGoal", s=w539, f=w538) -> (s? t:f=w533:T14)
        n178 = Select(t=T14."BumperShot", s=w532, f=w533) -> (s? t:f=w529:T14)
      }
      frame "LowGoal" {
        w544 = 1800.0 ("x")
        # "LowGoal. Readies shooters at 4000 RPMs; feeders remain still. Exits if shooters are running with in +-5% of correct speed and shooter button is pressed or to HighGoal if HighGoalButton is pressed."
        n179 = call "TOF.vi"("Delay (ms)"=u32 3000, "Input"=w559) -> ("Output"=w558:bool)  [unwired: 9 in]
        n180 = global read "Robot Global Data.vi" "TeleopButtonShooterAngleHighGoal"() -> (w568:bool)
        n181 = Greater?(x=w545, y=w544) -> (0:w546:bool)
        n182 = Greater?(x=w548, y=w544) -> (0:w547:bool)
        n183 = global read "Robot Global Data.vi" "TeleopButtonBumperShot"() -> (w566:bool)
        n184 = Select(t=T14."HighGoal", s=w568, f=w567) -> (s? t:f=w565:T14)
        n185 = And(x=w547, y=w546) -> (x .and. y?=w550:bool)
        n186 = Select(t=T14."BumperShot", s=w566, f=w565) -> (s? t:f=w564:T14)
        n187 = And(x=w550, y=w549) -> (x .and. y?=w551:bool)
        n188 = Select(t=T14."Shoot", s=w551, f=w564) -> (s? t:f=w560:T14)
        n189 = Select(t=w560, s=w558, f=T14."Empty") -> (s? t:f=w561:T14)
        n190 = global read "Robot Global Data.vi" "LowGoalSpeed"() -> (w553:dbl)
      }
      frame "HighGoal" {
        (unwired) u32 3000 ("Delay (ms)")
        (unwired) 0.0
        # "HighGoal. Readies shooters at 6000 RPMs; feeders remain still. Exits if shooters are running with in +-5% of correct speed and shooter button is pressed or to LowGoal if LowGoalButton is pressed."
        n191 = Absolute Value(x=w569) -> (abs(x)=w612:dbl)
        n192 = call "TOF.vi"("Delay (ms)"=u32 3000, "Input"=w595) -> ("Output"=w596:bool)  [unwired: 9 in]
        n193 = Absolute Value(x=w611) -> (abs(x)=w610:dbl)
        n194 = global read "Robot Global Data.vi" "HighGoalSpeed"() -> (w573:dbl)
        n195 = global read "Robot Global Data.vi" "Low Goal Shooter Button"() -> (w605:bool)
        n196 = global read "Robot Global Data.vi" "HighGoalShootPosition"() -> (w576:dbl)
        n197 = global read "Robot Global Data.vi" "TeleopButtonBumperShot"() -> (w603:bool)
        n198 = Absolute Value(x=w573) -> (abs(x)=w570:dbl)
        n199 = Absolute Value(x=w573) -> (abs(x)=w571:dbl)
        n200 = global read "Robot Global Data.vi" "ShooterAngleOffset"() -> (w580:dbl)
        n201 = Multiply(x=1.03, y=w571) -> (x*y=w609:dbl)
        n202 = Multiply(x=0.97, y=w570) -> (x*y=w606:dbl)
        n203 = Equal?(x=w584, y=T13."EmergencyManualControl") -> (x = y?=w585:bool)
        n204 = In Range and Coerce(upper limit=w609, x=w612, lower limit=w606) -> (In Range?=w614:bool)  [unwired: 1 out]
        n205 = In Range and Coerce(upper limit=w609, x=w610, lower limit=w606) -> (In Range?=w613:bool)  [unwired: 1 out]
        n206 = Select(t=T14."LowGoal", s=w605, f=w604) -> (s? t:f=w602:T14)
        n207 = Add(x=w576, y=0.2) -> (x+y=w578:dbl)
        n208 = Subtract(x=w576, y=0.2) -> (x-y=w577:dbl)
        n209 = Select(t=T14."BumperShot", s=w603, f=w602) -> (s? t:f=w601:T14)
        n210 = Add(x=w580, y=w578) -> (x+y=w581:dbl)
        n211 = Add(x=w580, y=w577) -> (x+y=w579:dbl)
        n212 = And(x=w614, y=w613) -> (x .and. y?=w592:bool)
        n213 = In Range and Coerce(upper limit=w581, x=w587, lower limit=w579) -> (In Range?=w586:bool)  [unwired: 1 out]
        n214 = And(x=w592, y=w615) -> (x .and. y?=w589:bool)
        n215 = Or(x=w585, y=w586) -> (x .or. y?=w582:bool)
        n216 = And(x=w582, y=w589) -> (x .and. y?=w588:bool)
        n217 = Select(t=T14."Shoot", s=w588, f=w601) -> (s? t:f=w597:T14)
        n218 = Select(t=w597, s=w596, f=T14."Empty") -> (s? t:f=w598:T14)
      }
      frame "BumperShot" {
        # "BumperShot"
        n219 = Absolute Value(x=w636) -> (abs(x)=w643:dbl)
        n220 = call "TOF.vi"("Delay (ms)"=u32 3000, "Input"=w627) -> ("Output"=w628:bool)  [unwired: 9 in]
        n221 = global read "Robot Global Data.vi" "BumperShotSpeed"() -> (w618:dbl)
        n222 = global read "Robot Global Data.vi" "Low Goal Shooter Button"() -> (w638:bool)
        n223 = global read "Robot Global Data.vi" "TeleopButtonShooterAngleHighGoal"() -> (w633:bool)
        n224 = Absolute Value(x=w637) -> (abs(x)=w644:dbl)
        n225 = Absolute Value(x=w618) -> (abs(x)=w616:dbl)
        n226 = Multiply(x=1.05, y=w616) -> (x*y=w642:dbl)
        n227 = Multiply(x=0.95, y=w616) -> (x*y=w639:dbl)
        n228 = In Range and Coerce(upper limit=w642, x=w644, lower limit=w639) -> (In Range?=w646:bool)  [unwired: 1 out]
        n229 = In Range and Coerce(upper limit=w642, x=w643, lower limit=w639) -> (In Range?=w645:bool)  [unwired: 1 out]
        n230 = Select(t=T14."LowGoal", s=w638, f=w634) -> (s? t:f=w632:T14)
        n231 = Select(t=T14."HighGoal", s=w633, f=w632) -> (s? t:f=w631:T14)
        n232 = And(x=w646, y=w645) -> (x .and. y?=w620:bool)
        n233 = And(x=w620, y=w635) -> (x .and. y?=w619:bool)
        n234 = Select(t=T14."Shoot", s=w619, f=w631) -> (s? t:f=w624:T14)
        n235 = Select(t=w624, s=w628, f=T14."Empty") -> (s? t:f=w629:T14)
      }
      frame "Shoot" {
        # "Shoot. Maintains shooters at current set rate and sets feeders at -.5 . Exits to dwell if photoeye has been false for 1 second (i.e. ball has been fired)."
        n236 = Select(t=T14."Dwell", s=w647, f=w651) -> (s? t:f=w656:T14)
        n237 = Select(t=WPI_SolenoidValue."On" ("Value"), s=w648, f=WPI_SolenoidValue."Off") -> (s? t:f=w650:T18)
      }
      frame "Dwell" {
        # "Dwell. Maintains shooters at current speed and sets feeders to 1000 (which should be current speed). Exits to empty after 2 seconds."
        n238 = Select(t=T14."Empty", s=w660, f=w663) -> (s? t:f=w662:T14)
      }
    }
    n239 = case "Shooter Angle State Machine" shown="\"Hold\"" w166 {
      selector: w166 -> [_ w404 _ _ _ w462 _ w478]
      tunnel: [WPI_CANTalonSRX_APIControlMode."Percent VBus" ("Control Mode") WPI_CANTalonSRX_APIControlMode."Percent VBus" ("Control Mode") WPI_CANTalonSRX_APIControlMode."Position" ("Control Mode") WPI_CANTalonSRX_APIControlMode."Position" ("Control Mode") WPI_CANTalonSRX_APIControlMode."Position" ("Control Mode") WPI_CANTalonSRX_APIControlMode."Position" ("Control Mode") WPI_CANTalonSRX_APIControlMode."Position" ("Control Mode") WPI_CANTalonSRX_APIControlMode."Percent VBus" ("Control Mode")] -> w267
      tunnel: [0.1 ("Output") -0.25 ("Output") 2.0 ("Output") w422 w432 w450 w471 w476] -> w40
      tunnel: [T13."Reset" w405 T13."Hold" T13."Hold" T13."Hold" w452 T13."Hold" w478] -> w259
      tunnel: w147 -> [_ _ w413 _ _ _ _ _]
      tunnel: w216 -> [_ _ _ _ _ w454 _ _]
      tunnel: w255 -> [_ _ _ _ _ _ _ w477]
      tunnel: w160 -> [_ w406 _ _ _ _ _ _]
      frame "ResetForward" {
        # "ResetForward"
      }
      frame "ResetBack", Default {
        (unwired) TRUE
        # "ResetBack"
        n240 = Select(t=T13."Reset", s=w406, f=w404) -> (s? t:f=w405:T13)
      }
      frame "Reset" {
        # "Reset"
        n241 = call <vilib>:"WPI_CANTalonSRX_SetSensorPosition.vi"("New Sensor Position"=0.0, "CAN Talon SRX Ref"=w413) -> ()  [unwired: 8 in, 2 out]
      }
      frame "HighGoal" {
        # "HighGoal"
        n242 = global read "Robot Global Data.vi" "IsCompBot"() -> (w418:bool)
        n243 = global read "Robot Global Data.vi" "ShooterAngleOffset"() -> (w421:dbl)
        n244 = global read "Robot Global Data.vi" "Y Axis Offset"() -> (w415:dbl)
        n245 = Select(t="High Goal Shooter Angle\n(Competition Bot)", s=w418, f="High Goal Shooter Angle\n(Practice Bot)") -> (s? t:f=w420:dbl)
        n246 = Add(x=w420, y=w421) -> (x+y=w416:dbl)
        n247 = Add(x=w416, y=w415) -> (x+y=w414:dbl)
        n248 = Multiply(x=w414, y=4096.0) -> (x*y=w422:dbl)
        n249 = global write "Robot Global Data.vi" "HighGoalShootPosition"(w414) -> ()
      }
      frame "LowGoal" {
        # "LowGoal"
        n250 = global read "Robot Global Data.vi" "IsCompBot"() -> (w427:bool)
        n251 = global read "Robot Global Data.vi" "ShooterAngleOffset"() -> (w431:dbl)
        n252 = Select(t="Low Goal Shooter Angle\n(Competition Bot)", s=w427, f="Low Goal Shooter Angle\n(Practice Bot)") -> (s? t:f=w426:dbl)
        n253 = Add(x=w426, y=w431) -> (x+y=w430:dbl)
        n254 = Multiply(x=w430, y=4096.0) -> (x*y=w432:dbl)
      }
      frame "Hold" {
        w444 = 4096.0 ("x")
        # "Hold"
        n255 = global read "Robot Global Data.vi" "Low Goal Shooter Button"() -> (w463:bool)
        n256 = global read "Robot Global Data.vi" "TeleopButtonShooterAngleHighGoal"() -> (w461:bool)
        n257 = global read "Robot Global Data.vi" "AutoShooterAngleSetHeight"() -> (w447:dbl)
        n258 = global read "Robot Global Data.vi" "IsCompBot"() -> (w440:bool)
        n259 = global read "Robot Global Data.vi" "ShooterAngleOffset"() -> (w446:dbl)
        n260 = global read "Robot Global Data.vi" "TeleopButtonRollerPickupBall"() -> (w438:bool)
        n261 = global read "Robot Global Data.vi" "TeleopButtonBumperShot"() -> (w458:bool)
        n262 = global read "Robot Global Data.vi" "TeleopButtonLowBar"() -> (w437:bool)
        n263 = Select(t="Pickup Ball Shooter Angle\n(Competition Bot)", s=w440, f="Pickup Ball Shooter Angle\n(Practice Bot)") -> (s? t:f=w439:dbl)
        n264 = Select(t=T13."LowGoal", s=w463, f=w462) -> (s? t:f=w460:T13)
        n265 = Select(t=T13."HighGoal", s=w461, f=w460) -> (s? t:f=w459:T13)
        n266 = Add(x=w447, y=w446) -> (x+y=w445:dbl)
        n267 = Add(x=w439, y=w446) -> (x+y=w451:dbl)
        n268 = global read "Robot Global Data.vi" "AutoShooterArmAngleControl"() -> (w449:bool)
        n269 = Multiply(x=w445, y=w444) -> (x*y=w443:dbl)
        n270 = Multiply(x=w444, y=w451) -> (x*y=w453:dbl)
        n271 = Or(x=w438, y=w437) -> (x .or. y?=w436:bool)
        n272 = Select(t=T13."BumperShot", s=w458, f=w459) -> (s? t:f=w452:T13)
        n273 = Select(t=w453, s=w436, f=w454) -> (s? t:f=w448:dbl)
        n274 = Select(t=w443, s=w449, f=w448) -> (s? t:f=w450:dbl)
      }
      frame "BumperShot" {
        # "BumperShot"
        n275 = global read "Robot Global Data.vi" "IsCompBot"() -> (w466:bool)
        n276 = global read "Robot Global Data.vi" "ShooterAngleOffset"() -> (w470:dbl)
        n277 = Select(t="Bumper Shot Shooter Angle\n(Competition Bot)", s=w466, f="Bumper Shot Shooter Angle\n(Practice Bot)") -> (s? t:f=w465:dbl)
        n278 = Add(x=w465, y=w470) -> (x+y=w469:dbl)
        n279 = Multiply(x=4096.0 ("y"), y=w469) -> (x*y=w471:dbl)
      }
      frame "EmergencyManualControl" {
        n280 = Multiply(x=w477, y=0.4) -> (x*y=w476:dbl)
      }
    }
    n281 = Multiply(x=w82, y=4096.0) -> (x*y=w81:dbl)
    n282 = Equal?(x=w74, y=w81) -> (x = y?=w79:bool)
    n283 = feedback-in #1(w74) -> ()
    n284 = feedback #1() -> (w75:dbl)  [unwired: 1 in]
    n285 = Not Equal?(x=w75, y=w74) -> (x != y?=w72:bool)
    n286 = Not Equal To 0?(x=w181) -> (x != 0?=w131:bool)
    n287 = case shown="\"Set LowBar\"" w73 {
      selector: w73 -> [w308 _ _]
      tunnel: w79 -> [w305 _ _]
      tunnel: [w307 enum16{"Hold", "Set LowBar", "Set Normal"}."Hold" ("t") enum16{"Hold", "Set LowBar", "Set Normal"}."Hold" ("t")] -> w78
      tunnel: w77 -> [_ _ w327]
      tunnel: w76 -> [_ w318 w321]
      tunnel: w42 -> [_ w319 _]
      tunnel: w72 -> [w306 _ _]
      frame "Hold", Default {
        n288 = Select(t=enum16{"Hold", "Set LowBar", "Set Normal"}."Set LowBar", s=w305, f=enum16{"Hold", "Set LowBar", "Set Normal"}."Set Normal") -> (s? t:f=w309:enum16{"Hold", "Set LowBar", "Set Normal"})
        n289 = Select(t=w309, s=w306, f=w308) -> (s? t:f=w307:enum16{"Hold", "Set LowBar", "Set Normal"})
      }
      frame "Set LowBar" {
        n290 = Unbundle(w319) -> ("Wonder Arm P 2"=w317:dbl, "Wonder Arm I 2"=w316:dbl, "Wonder Arm D 2"=w315:dbl, "Wonder Arm F 2"=w314:dbl, "Wonder Arm I-Zone 2"=w313:dbl)
        n291 = call <vilib>:"WPI_CANTalonSRX_SetPID.vi"("CAN Talon SRX Ref"=w318, "P"=w317, "I"=w316, "D"=w315, "F"=w314, "I Zone"=w313) -> ()  [unwired: 8 in, 2 out]
      }
      frame "Set Normal" {
        n292 = Unbundle(w327) -> ("Wonder Arm P"=w326:dbl, "Wonder Arm I"=w325:dbl, "Wonder Arm D"=w324:dbl, "Wonder Arm F"=w323:dbl, "Wonder Arm I-Zone"=w322:dbl)
        n293 = call <vilib>:"WPI_CANTalonSRX_SetPID.vi"("CAN Talon SRX Ref"=w321, "P"=w326, "I"=w325, "D"=w324, "F"=w323, "I Zone"=w322) -> ()  [unwired: 8 in, 2 out]
      }
    }
    n294 = Compound Arithmetic op=AND(w55, w54, w131) -> (w130:bool)
    n295 = call "TON.vi"("Delay (ms)"=u32 2000, "Input"=w130) -> ("Output"=w180:bool)  [unwired: 9 in]
    n296 = global write "Robot Global Data.vi" "IsStalled"(w180) -> ()
    n297 = global read "Robot Global Data.vi" "IsAutoTargeting"() -> (w86:bool)
    n298 = Equal?(x=w236, y=T12."EmergencyManualControl") -> (x = y?=w249:bool)
    n299 = Equal?(x=w235, y=WPI_CANTalonSRX_APIControlMode."Percent VBus") -> (x = y?=w233:bool)
    n300 = Multiply(x="Suck Wheel Speed", y=0.9) -> (x*y=w111:dbl)
    n301 = global read "Robot Global Data.vi" "Wonder Arm Vision Position"() -> (w50:dbl)
    n302 = global read "Robot Global Data.vi" "ShooterWheelCountsPerRevolution"() -> (w146:dbl)
    n303 = Multiply(x=w50, y=4096.0) -> (x*y=w85:dbl)
    n304 = Select(t=w85, s=w86, f=w74) -> (s? t:f=w83:dbl)
    n305 = call <vilib>:"WPI_CANTalonSRX_ChangeMode.vi"("Output"=w83, "Control Mode"=w235, "CAN Talon SRX Ref"=w76) -> ()  [unwired: 7 in, 2 out]
    n306 = Divide(x=w83, y=4096.0) -> (x/y=w99:dbl)
    n307 = global write "Robot Global Data.vi" "DashboardRollerArmDesired"(w99) -> ()
    n308 = Select(t=w145, s=w233, f=w83) -> (s? t:f=w261:dbl)
    n309 = Greater?(x=w111, y=w94) -> (0:w110:bool)
    n310 = And(x=w114, y=w110) -> (x .and. y?=w113:bool)
    n311 = Or(x=w249, y=w113) -> (x .or. y?=w248:bool)
    n312 = Select(t=0.5, s=w248, f=0.0) -> (s? t:f=w253:dbl)
    n313 = call <vilib>:"WPI_MotorControlSetOutput.vi"("Output"=w253, "MotorControlDevRef"=w188) -> ()  [unwired: 7 in, 3 out]
    n314 = call <vilib>:"WPI_CANTalonSRX_ChangeMode.vi"("Output"=w40, "Control Mode"=w267, "CAN Talon SRX Ref"=w147) -> ()  [unwired: 7 in, 2 out]
    n315 = global write "Robot Global Data.vi" "DashboardShooterAngleDesired"(w40) -> ()
    n316 = Divide(x=w146, y=600.0) -> (x/y=w290:dbl)
    n317 = global read "Robot Global Data.vi" "AutoShooterSpeedControl"() -> (w171:bool)
    n318 = global read "Robot Global Data.vi" "AutoShooterSpeedValue"() -> (w102:dbl)
    n319 = Divide(x=w102, y=1.375) -> (x/y=w100:dbl)
    n320 = global read "Robot Global Data.vi" "SuckButton"() -> (w115:bool)
    n321 = global read "Robot Global Data.vi" "SuckSpeed"() -> (w116:dbl)
    n322 = global read "Robot Global Data.vi" "ShooterWheelCountsPerRevolution"() -> (w129:dbl)
    n323 = Select(t=w116, s=w115, f=w117) -> (s? t:f=w118:dbl)
    n324 = global read "Robot Global Data.vi" "IsStalled"() -> (w176:bool)
    n325 = Select(t=w100, s=w171, f=w118) -> (s? t:f=w170:dbl)
    n326 = Select(t=0.0, s=w176, f=w170) -> (s? t:f=w87:dbl)
    n327 = global write "Robot Global Data.vi" "ShooterMotorRightDesiredRPM"(w87) -> ()
    n328 = Equal?(x=w87, y=w53) -> (x = y?=w274:bool)
    n329 = Multiply(x=w87, y=w290) -> (x*y=w189:dbl)
    n330 = Multiply(x=1.375, y=w87) -> (x*y=w88:dbl)
    n331 = Not(x=w274) -> (.not. x?=w134:bool)
    n332 = Select(t=0.0, s=w176, f=w170) -> (s? t:f=w90:dbl)
    n333 = global write "Robot Global Data.vi" "DesiredRPM1"(w90) -> ()
    n334 = Multiply(x=1.375, y=w90) -> (x*y=w91:dbl)
    n335 = global write "Robot Global Data.vi" "DashboardWheelTwoDesired"(w91) -> ()
    n336 = global read "Robot Global Data.vi" "IsStalled"() -> (w132:bool)
    n337 = Equal To 0?(x=w90) -> (x = 0?=w272:bool)
    n338 = Not Equal?(x=w191, y=w90) -> (x != y?=w136:bool)
    n339 = Divide(x=w129, y=600.0) -> (x/y=w277:dbl)
    n340 = Multiply(x=w90, y=w277) -> (x*y=w190:dbl)
    n341 = Or(x=w136, y=w132) -> (x .or. y?=w135:bool)
    n342 = global write "Robot Global Data.vi" "DashboardWheelOneDesired"(w88) -> ()
    n343 = case shown="True" w135 {
      tunnel: w273 -> [w480 w488]
      tunnel: w272 -> [_ w483]
      tunnel: [w480 w484] -> w271
      tunnel: w132 -> [_ w482]
      frame False {
      }
      frame True {
        n344 = Or(x=w483, y=w482) -> (x .or. y?=w481:bool)
        n345 = Select(t=WPI_CANTalonSRX_APIControlMode."Percent VBus" ("Control Mode"), s=w481, f=WPI_CANTalonSRX_APIControlMode."Speed") -> (s? t:f=w486:T11)
        n346 = call <vilib>:"WPI_CANTalonSRX_ChangeMode.vi"("Control Mode"=w486, "CAN Talon SRX Ref"=w488) -> ("CAN Talon SRX Ref"=w484:T5)  [unwired: 8 in, 1 out]
      }
    }
    n347 = Or(x=w134, y=w132) -> (x .or. y?=w133:bool)
    n348 = Equal To 0?(x=w87) -> (x = 0?=w270:bool)
    n349 = call-poly <vilib>:"WPI_SolenoidSet.vi"("Value"=w67, "SolenoidDevRef"=w68) -> ()  [unwired: 8 in, 2 out]
    n350 = case shown="True" w133 {
      tunnel: [w489 w497] -> w275
      tunnel: w276 -> [w489 w496]
      tunnel: w270 -> [_ w492]
      tunnel: w132 -> [_ w491]
      frame False {
      }
      frame True {
        n351 = Or(x=w492, y=w491) -> (x .or. y?=w490:bool)
        n352 = Select(t=WPI_CANTalonSRX_APIControlMode."Percent VBus" ("Control Mode"), s=w490, f=WPI_CANTalonSRX_APIControlMode."Speed") -> (s? t:f=w494:T11)
        n353 = call <vilib>:"WPI_CANTalonSRX_ChangeMode.vi"("Control Mode"=w494, "CAN Talon SRX Ref"=w496) -> ("CAN Talon SRX Ref"=w497:T5)  [unwired: 8 in, 1 out]
      }
    }
    n354 = call-poly <vilib>:"WPI_SolenoidSet.vi"("Value"=w56, "SolenoidDevRef"=w108) -> ()  [unwired: 8 in, 2 out]
    n355 = global write "Robot Global Data.vi" "BallHaloCylinder"(w56) -> ()
    n356 = global write "Robot Global Data.vi" "BallShooterCylinder"(w67) -> ()
    n357 = call <vilib>:"WPI_MotorControlSetOutput.vi"("Output"=w190, "MotorControlDevRef"=w271) -> ()  [unwired: 7 in, 3 out]
    n358 = global read "Robot Global Data.vi" "AutoArmControl"() -> (w39:bool)
    n359 = call <vilib>:"WPI_MotorControlSetOutput.vi"("Output"=w189, "MotorControlDevRef"=w275) -> ()  [unwired: 7 in, 3 out]
  }
